vi "1C.1 Camera - Find Marker.vi"(8 "error in":errorcluster, 9 "Minimum Match Score (650)":sgl=650.0, 10 "marker template relative path":string="..\\1C Tracking Patterns\\4.5mm-BowMarker.png", 11 "Image In":T3(plugin-control)) -> (0 "error out":errorcluster, 1 "Best Match Position":cluster{"x":sgl, "y":sgl}, 2 "Best Match Heading":T1 format="%05.1f", 3 "Image Out":T3, 5 "Marker found?":T2)   [LabVIEW 2011]
doc: "Finds a glyph in an image, and returns: a boolean of whether the glyph could be found, the location of the best match in the image, and its rotation from the glyph template.\n\nTODO: test this with real markers and images.\n\nCoders: Cory, Gray and Jason\n\nRationale: For the Small RC platform, this is the VI that actually locates the two markers on the boat in an image, and returns their positions if they were found."
uses:
  <vilib>/vision/Image Controls.llb/IMAQ Image.ctl
  2-RIO/2 Typedefs/indicator LED.ctl
  2-RIO/2 Typedefs/heading.ctl
  <vilib>/vision/NI_Vision_Development_Module.lvlib
panel:
  in  "File Path":path
  out "Best Match":T4
  out "marker template absolute path":path
  out "Marker Template":T3(plugin-control)
  out "Matches":T5(array[cluster]) {"Bounding Box"."y" format="%.2f"; "Bounding Box"."x" format="%.2f"; "Position"."y" format="%.2f"; "Position"."x" format="%.2f"; "Score" format="%.2f"; "Scale" format="%.2f"; "Angle" format="%.2f"}
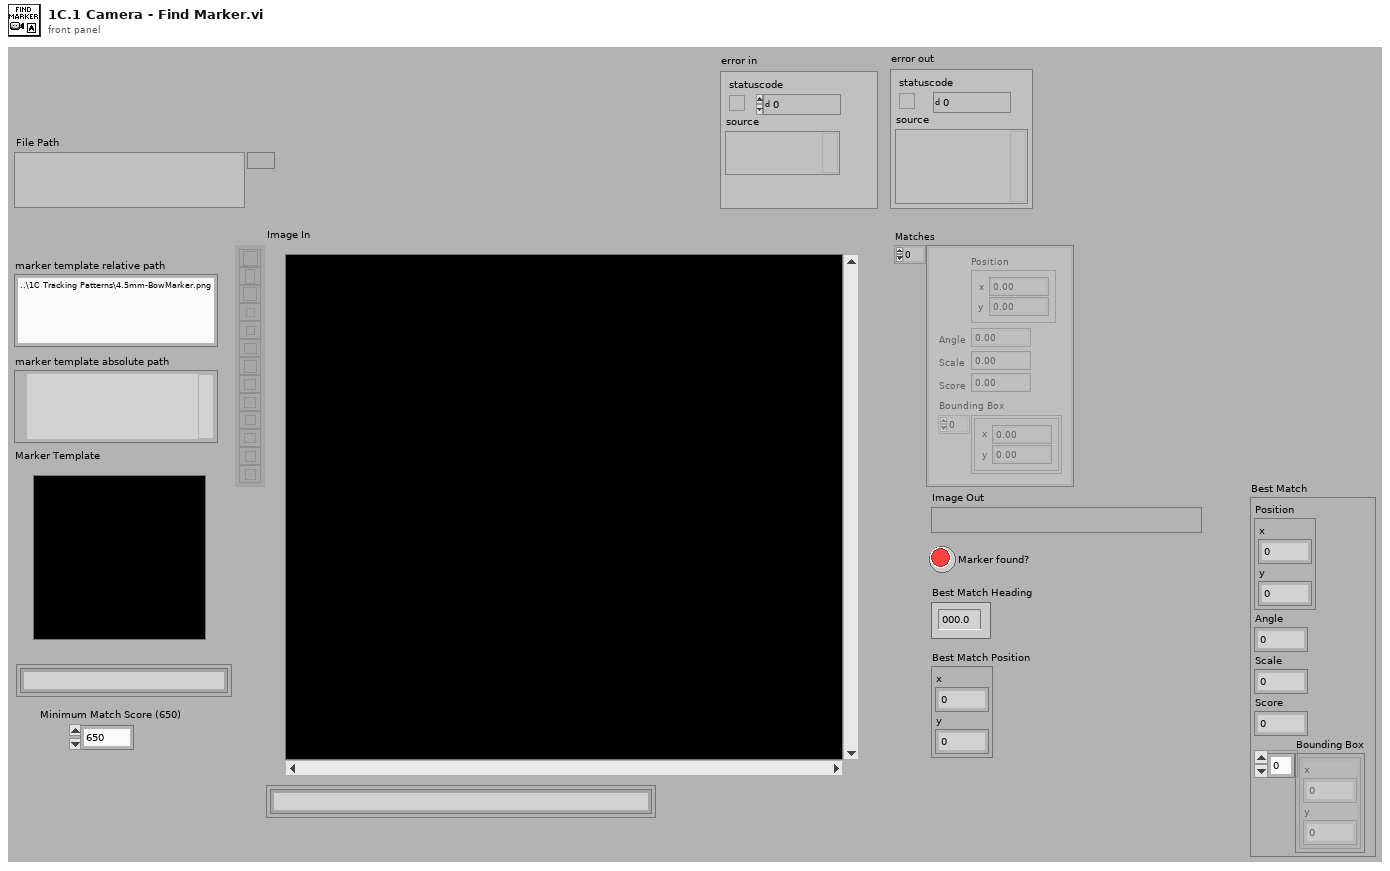
[diagram p1: front panel]
types:
  T1 = typedef "heading.ctl" = dbl
  T2 = typedef "indicator LED.ctl" = bool
  T3 = typedef "IMAQ Image.ctl" = refnum<image>
  T4 = cluster{"Position":cluster{"x":sgl, "y":sgl}, "Angle":sgl, "Scale":sgl, "Score":sgl, "Bounding Box":cluster{"x":sgl, "y":sgl}[]}
  T5 = cluster{"Position":cluster{"x":sgl, "y":sgl}, "Angle":sgl, "Scale":sgl, "Score":sgl, "Bounding Box":cluster{"x":sgl, "y":sgl}[]}[]
  T6 = typedef "Image Type" = u32
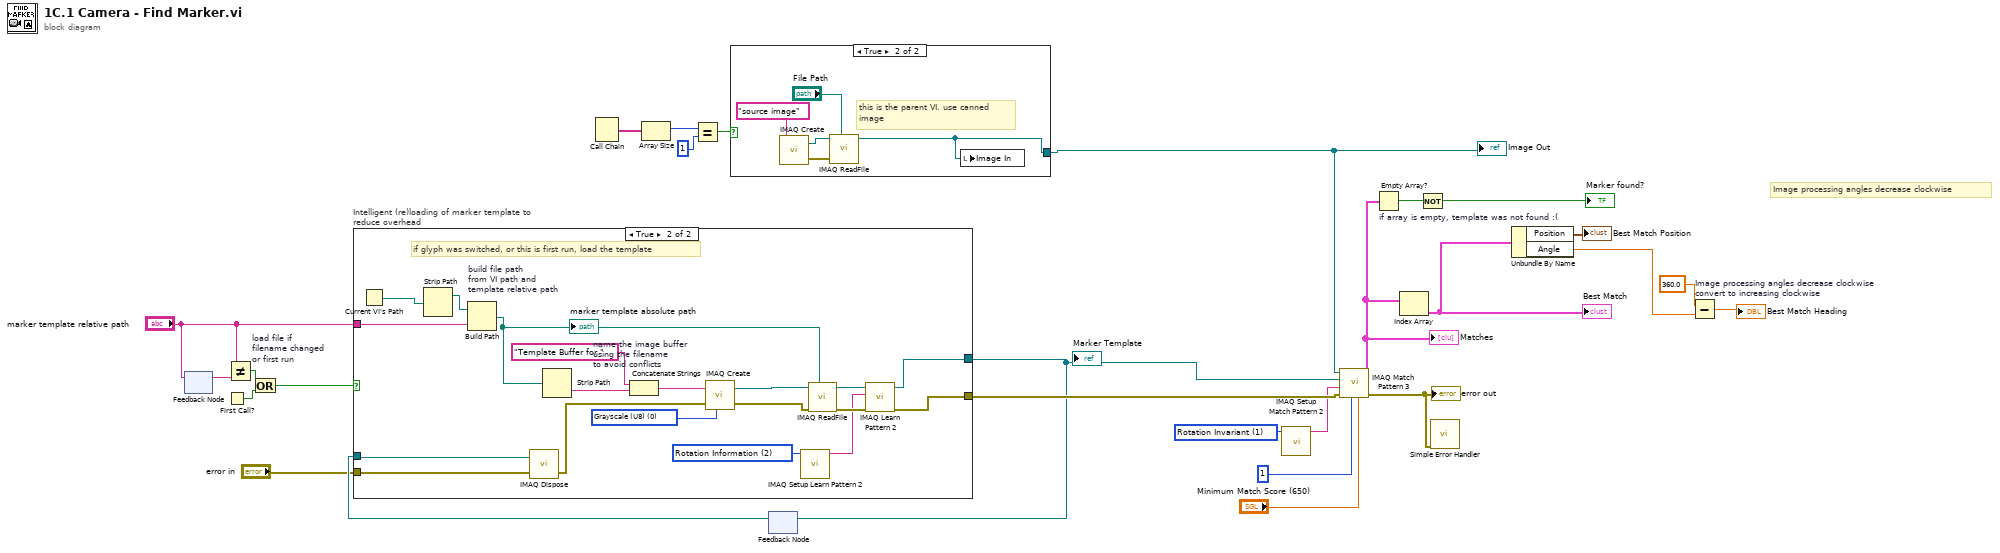
[diagram p0: block diagram]
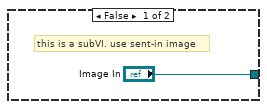
[diagram p2: hidden frame]
diagram:
  w11 = u16 1 items=["Shift Invariant", "Rotation Invariant"] ("Match Mode 2")
  # "Image processing angles decrease clockwise"
  n1 = feedback-in #1("marker template relative path") -> ()
  n2 = feedback #1() -> (w26:string)  [unwired: 1 in]
  n3 = First Call?() -> (First Call?: T/F=w23:bool)
  n4 = Not Equal?(x="marker template relative path", y=w26) -> (x != y?=w24:bool)
  n5 = Or "load file if\nfilename changed\nor first run"(x=w24, y=w23) -> (x .or. y?=w12:bool)
  n6 = Call Chain() -> (call chain=w3:string[])
  n7 = Array Size(array=w3) -> (size(s)=w5:i32)
  n8 = Equal?(x=w5, y=1) -> (x = y?=w2:bool)
  n9 = case shown="True" w2 {
    tunnel: ["Image In" w31] -> w1
    frame False {
      # "this is a subVI. use sent-in image"
    }
    frame True {
      # "this is the parent VI. use canned\nimage"
      n10 = call "IMAQ Create"("Image Name"="source image") -> ("New Image"=w33:T3, "error out"=w32:errorcluster)  [unwired: 4 in]
      n11 = call "IMAQ ReadFile"("File Path"="File Path", "error in (no error)"=w32, "Image"=w33) -> ("Image Out"=w31:T3)  [unwired: 4 in, 4 out]
      n12 = local write "Image In"(w31) -> ()
    }
  }
  "Image Out" <- w1
  n13 = feedback #2() -> (w25:T3)  [unwired: 1 in]
  n14 = case "Intelligent (re)loading of marker template to reduce overhead" shown="True" w12 {
    tunnel: [w35 w40] -> w13
    tunnel: "marker template relative path" -> [_ w50]
    tunnel: w25 -> [w35 w49]
    tunnel: [w34 w38] -> w18
    tunnel: "error in" -> [w34 w47]
    frame False {
      # "if the path has not changed,\njust keep the same template from last time"
    }
    frame True {
      w37 = u16 2 items=["All", "Shift Information", "Rotation Information"] ("Learn Mode")
      w53 = T6 0 items=["Grayscale (U8)", "Grayscale (I16)", "Grayscale (SGL)", "Complex (CSG)", "RGB (U32)", "HSL (U32)", "RGB (U64)", "Grayscale (U16)"] ("Image Type")
      # "if glyph was switched, or this is first run, load the template"
      n15 = Current VI's Path() -> (path=w52:path)
      n16 = Strip Path(path=w52) -> (stripped path=w51:path)  [unwired: 1 out]
      n17 = Build Path "build file path\nfrom VI path and \ntemplate relative path"(base path=w51, name or relative path=w50) -> (appended path=w44:path)
      "marker template absolute path" <- w44
      n18 = call "IMAQ Dispose"("Image"=w49, "error in (no error)"=w47) -> ("error out"=w46:errorcluster)  [unwired: 4 in]
      n19 = Strip Path(path=w44) -> (name=w42:string)  [unwired: 1 out]
      n20 = Concatenate Strings "name the image buffer\nusing the filename\nto avoid conflicts"("Template Buffer for " ("Image Name"), w42) -> (w45:string)
      n21 = call "IMAQ Create"("Image Name"=w45, "Image Type"=w53, "error in (no error)"=w46) -> ("New Image"=w54:T3, "error out"=w48:errorcluster)  [unwired: 2 in]
      n22 = call "IMAQ Setup Learn Pattern 2"("Learn Mode"=w37) -> ("Learn Pattern Setup Data"=w36:string)  [unwired: 9 in, 1 out]
      n23 = call "IMAQ ReadFile"("File Path"=w44, "error in (no error)"=w48, "Image"=w54) -> ("error out"=w39:errorcluster, "Image Out"=w41:T3)  [unwired: 4 in, 3 out]
      n24 = call "IMAQ Learn Pattern 2"("error in (no error)"=w39, "Learn Pattern Setup Data"=w36, "Image"=w41) -> ("error out"=w38:errorcluster, "Template Image Out"=w40:T3)  [unwired: 7 in]
    }
  }
  "Marker Template" <- w13
  n25 = feedback-in #2(w13) -> ()
  n26 = call "IMAQ Setup Match Pattern 2"("Match Mode"=w11) -> ("Match Pattern Setup Data"=w8:string)  [unwired: 9 in, 1 out]
  n27 = call "IMAQ Match Pattern 3"("Minimum Match Score"="Minimum Match Score (650)", "Number of Matches Requested"=1, "error in (no error)"=w18, "Match Pattern Setup Data"=w8, "Template Image"=w13, "Image"=w1) -> ("error out"=w6:errorcluster, "Matches"=w7:T5)  [unwired: 3 in, 1 out]
  "Matches" <- w7
  "error out" <- w6
  n28 = Empty Array? "if array is empty, template was not found :("(array=w7) -> (empty?=w20:bool)
  n29 = Index Array(array=w7) -> (element=w22:T4)  [unwired: 1 in]
  "Best Match" <- w22
  n30 = Not(x=w20) -> (.not. x?=→"Marker found?":bool)
  n31 = call <vilib>:"Simple Error Handler.vi"("error in (no error)"=w6) -> ()  [unwired: 4 in, 5 out]
  n32 = Unbundle By Name(w22) -> ("Position"=→"Best Match Position":cluster{"x":sgl, "y":sgl}, "Angle"=w15:sgl)
  n33 = Subtract "Image processing angles decrease clockwise\nconvert to increasing clockwise"(x=sgl 360.0 ("y"), y=w15) -> (x-y=→"Best Match Heading":sgl)
